vi "loadDataNodeEnd.vi"(8 "error in (no error)":errorcluster, 10 "XML Refnum in":refnum<file>, 11 "Category in":refnum<class "Category.lvclass">) -> (0 "error out":errorcluster, 2 "XML Refnum out":refnum<file>, 3 "Category out":refnum<class "Category.lvclass">)   [LabVIEW 2013, in "Category.lvclass"]
doc: "Part of the file loading process. Occurs at the end of a node being loaded. Includes checking the end of the tag which has the format </tag>."
uses:
  Category.lvclass
  xCE/xceDataNode/xceDataNode.lvclass
  XML Parser/XML Parser.lvclass
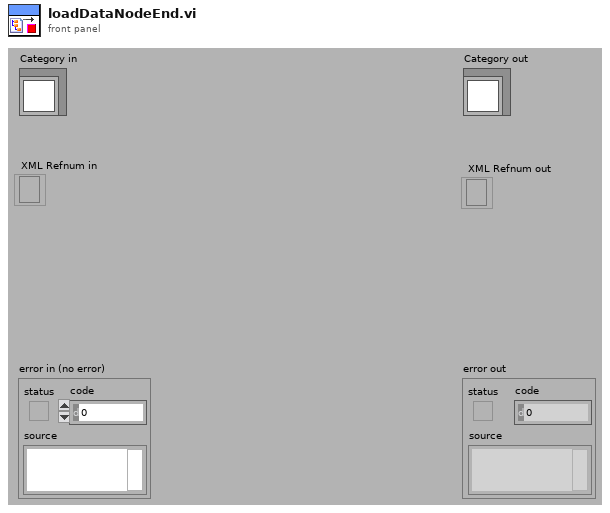
[diagram p1: front panel]
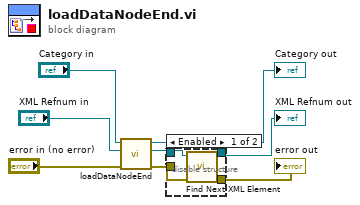
[diagram p0: block diagram]
diagram:
  n1 = call-parent "loadDataNodeEnd.vi"("error in (no error)"="error in (no error)", "XML Refnum in"="XML Refnum in", "xceDataNode in"="Category in") -> ("error out"=w1:errorcluster, "XML Refnum out"=w4:refnum<file>, "xceDataNode out"=→"Category out":refnum<class "Category.lvclass">)  [unwired: 6 in]
  n2 = disable-structure shown="Enabled" {
    disable-tunnel: w4 -> [w12 _]
    disable-tunnel: [w11 _] -> w3
    disable-tunnel: [w10 w13] -> w2
    disable-tunnel: w1 -> [w9 w13]
    frame Enabled {
      n3 = call "Find Next XML Element.vi"("error in (no error)"=w9, "XML Fine In"=w12) -> ("error out"=w10:errorcluster, "XML Fine Out"=w11:refnum<file>)  [unwired: 7 in, 1 out]
    }
    frame Disabled {
    }
  }
  "error out" <- w2
  "XML Refnum out" <- w3
